vi "UtilityLib.Operating System.vi"() -> (0 "Operation System":T1=enum."Windows")   [LabVIEW 2014, in "UtilityLib.lvlib"]
doc: "obtains the name of the operating system"
uses:
  UtilityLib.lvlib
  UtilityLib.Operation System.ctl
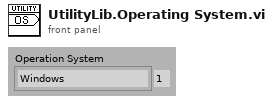
[diagram p1: front panel]
types:
  T1 = typedef "UtilityLib.lvlib/UtilityLib.Operation System.ctl" = enum16{"unknown", "Windows", "Embedded", "RT", "Mac", "Unix", "PocketPC"}
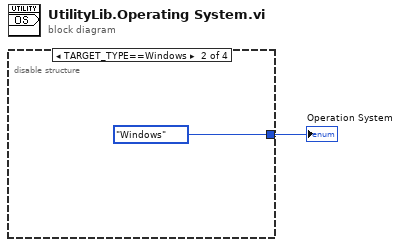
[diagram p0: block diagram]
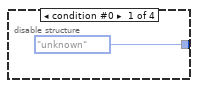
[diagram p2: hidden frame]
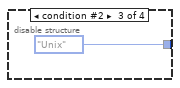
[diagram p3: hidden frame]
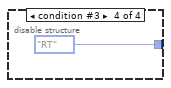
[diagram p4: hidden frame]
diagram:
  n1 = disable-structure shown="TARGET_TYPE==Windows" {
    disable-tunnel: [UtilityLib.Operation_System."unknown" ("Operation System") UtilityLib.Operation_System."Windows" ("Operation System") UtilityLib.Operation_System."Unix" ("Operation System") UtilityLib.Operation_System."RT" ("Operation System")] -> w1
    frame condition #0 {
    }
    frame condition #1 (active) {
    }
    frame condition #2 {
    }
    frame condition #3 {
    }
  }
  "Operation System" <- w1
